vi "Particle_Simulaation.vi"(8 "error in (no error)":errorcluster, 11 "Refnum in":T1) -> (0 "error out":errorcluster, 3 "Refnum out":T1)   [LabVIEW 2019]
uses:
  <vilib>/vision/Image Controls.llb/IMAQ Image.ctl
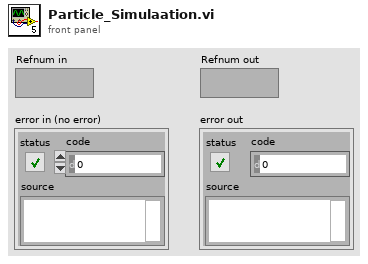
[diagram p1: front panel]
types:
  T1 = typedef "IMAQ Image.ctl" = refnum<image>
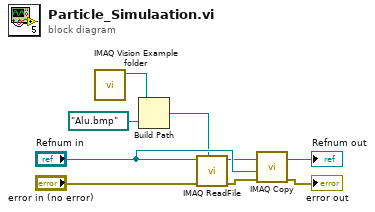
[diagram p0: block diagram]
diagram:
  n1 = call "IMAQ Vision Example folder.vi"() -> ("Example Image Path"=w2:path)  [unwired: 11 in]
  n2 = Build Path(base path=w2, name or relative path=path "Alu.bmp") -> (appended path=w4:path)
  n3 = call "IMAQ ReadFile"("File Path"=w4, "error in (no error)"="error in (no error)", "Image"="Refnum in") -> ("error out"=w6:errorcluster, "Image Out"=w5:T1)  [unwired: 4 in, 3 out]
  n4 = call "IMAQ Copy"("error in (no error)"=w6, "Image Dst"="Refnum in", "Image Src"=w5) -> ("error out"=→"error out":errorcluster, "Image Dst Out"=→"Refnum out":T1)  [unwired: 3 in]
